vi "[Callback]ListColColorUpdate.vi"(4 "User Parameter":variant, 5 "Event Data":T2, 6 "List":refnum<vi>, 7 "Event Common Data":cluster{"Source":T3, "Type":T4, "Time":u32} {"Source" items=["LabVIEW UI"=0, "ActiveX"=1, "User Event"=25]}) -> ()   [LabVIEW 2019]
uses:
  <vilib>/event_ctls.llb/eventsource.ctl
  <vilib>/event_ctls.llb/lveventtype.ctl
  <vilib>/Utility/miscctls.llb/LVPoint32TypeDef.ctl
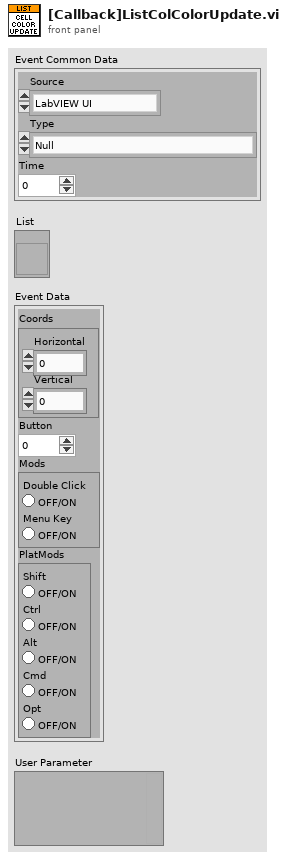
[diagram p1: front panel]
types:
  T1 = typedef "LVPoint32TypeDef.ctl" = cluster{"Horizontal":i32, "Vertical":i32}
  T2 = cluster{"Coords":T1, "Button":u16, "Mods":cluster{"Double Click":bool, "Menu Key":bool}, "PlatMods":cluster{"Shift":bool, "Ctrl":bool, "Alt":bool, "Cmd":bool, "Opt":bool}}
  T3 = typedef "eventsource.ctl" = u32
  T4 = typedef "lveventtype.ctl" = enum32{"Null", "Timeout", "Annotation Menu Selection", "Annotation Menu Selection?", "App Instance Close", "App Instance Close?", "Autoscale Range Change", "Bookmark Info Change", "Cell Edit", "Cell Edit?", "Cursor Grab", "Cursor Grab?", "Cursor Menu Selection", "Cursor Menu Selection?", "Cursor Move", "Cursor Release", "Data Change", "Direction Change", "Display State Change", "Drag Ended", "Drag Enter", "Drag Leave", "Drag Over", "Drag Source Update", "Drag Starting", "Drag Starting?", "Drop", "Exec State Change", "Key Down", "Key Down?", "Key Repeat", "Key Repeat?", "Key Up", "Listbox Double Click", "Menu Activation?", "Menu Selection (App)", "Menu Selection? (App)", "Menu Selection (User)", "Mouse Down", "Mouse Down?", "Mouse Enter", "Mouse Leave", "Mouse Move", "Mouse Up", "Mouse Wheel", "NI Security User Change (App)", "Pane Size", "Panel Close", "Panel Close?", "Panel Resize", "Plot Attribute Change", "Scale Range Change", "Shortcut Menu Activation?", "Shortcut Menu Selection (App)", "Shortcut Menu Selection? (App)", "Shortcut Menu Selection (User)", "Tree Double Click", "Tree Drag", "Tree Drag?", "Tree Drop", "Tree Drop?", "Tree Item Close", "Tree Item Close?", "Tree Item Open", "Tree Item Open?", "User Event", "Value Change"}
  T5 = typedef "LVRowAndColumnTypeDef.ctl" = cluster{"Row":i32, "Column":i32}
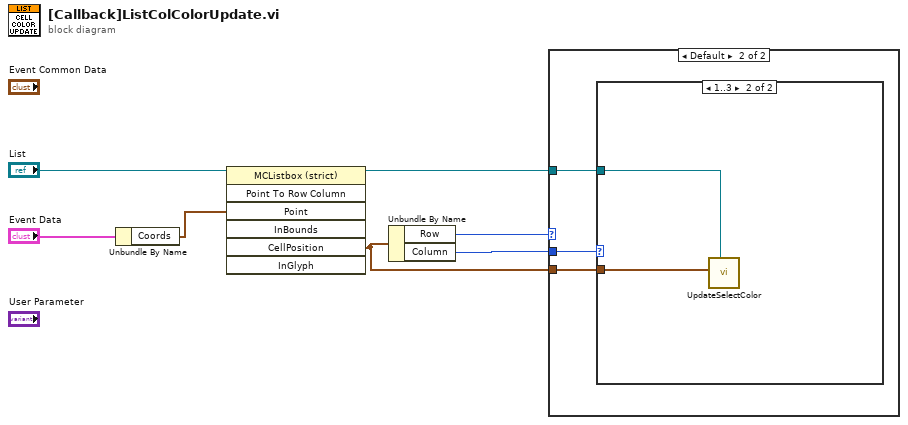
[diagram p0: block diagram]
diagram:
  n1 = Unbundle By Name("Event Data") -> ("Coords"=w5:T1)
  n2 = invoke class="MCListbox (strict)" method="Point To Row Column"(reference="List", "Point"=w5) -> (reference out=w1:refnum<vi>, "CellPosition"=w2:T5)  [unwired: 5 in, 5 out]
  n3 = Unbundle By Name(w2) -> ("Row"=w4:i32, "Column"=w3:i32)
  n4 = case shown="Default" w4 {
    tunnel: w3 -> [_ w10]
    tunnel: w2 -> [_ w9]
    tunnel: w1 -> [_ w8]
    frame -1 {
      # "No value is selected!"
    }
    frame Default {
      n5 = case shown="1..3" w10 {
        tunnel: w9 -> [_ w12]
        tunnel: w8 -> [_ w11]
        frame 0, Default {
          # "Click on the names' column!"
        }
        frame 1..3 {
          n6 = call "UpdateSelectColor.vi"("Available Points"=w11, "Available Points Idx"=w12) -> ()  [unwired: 9 in, 1 out]
        }
      }
    }
  }
